vi "LV SCISDK Read List Data.vi"(0 "Path":string, 1 "Buffer Size":u32=1, 2 "handle":u64, 3 "error in (no error)":errorcluster) -> (7 "error out":errorcluster, 8 "buffer out":T1, 9 "handle out":u64, 10 "function return":i32)   [LabVIEW 2021, in "SciSDK_Labview.lvlib"]
doc: "SCISDKLABVIEW_DLL_API int LV_SCISDK_ReadSpectrum(char* Path, TD_SPECTRUM* buffer, void* handle);"
uses:
  SciSDK_Labview.lvlib
panel:
  in  "buffer":T1={"magic"=0, "buffer_size"=0, "samples"=0, "valid_samples"=0, "channels"=0, "data"=[10, 100]}
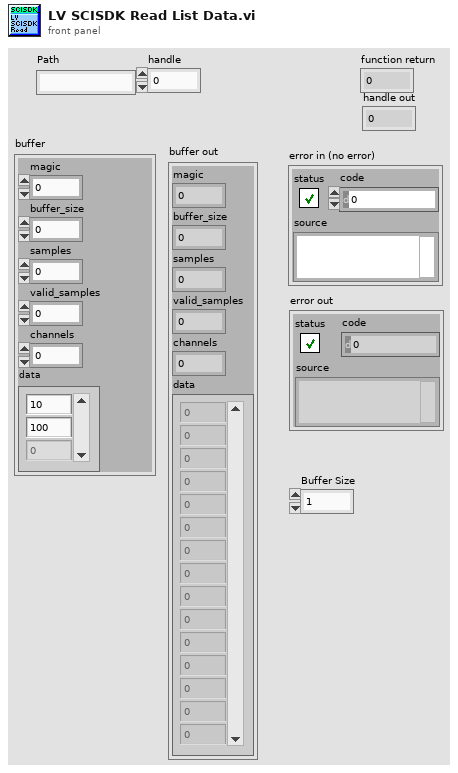
[diagram p1: front panel]
types:
  T1 = cluster{"magic":u32, "buffer_size":u32, "samples":u32, "valid_samples":u32, "channels":u32, "data":i8[]}
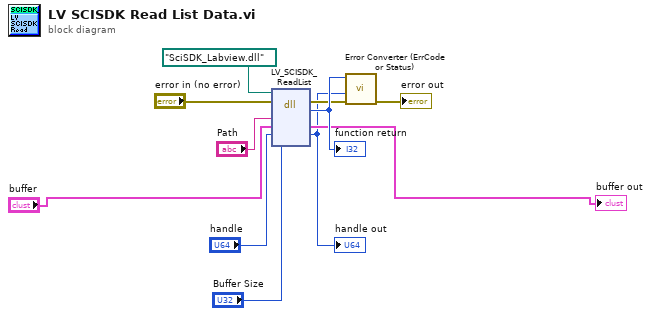
[diagram p0: block diagram]
diagram:
  n1 = dll-call lib="C:/git/scisdk/SciSDK_VC++/x64/Debug/SciSDK_Labview.dll" fn="LV_SCISDK_ReadList"(path in=path "SciSDK_Labview.dll", error in="error in (no error)", "Path"="Path", "buffer"="buffer", "handle"="handle", "buffer_size"="Buffer Size") -> (error out=w7:errorcluster, "return type"=w11:i32, "buffer"=→"buffer out":T1, "handle"=w1:u64)  [unwired: 3 in, 1 out]
  "function return" <- w11
  "handle out" <- w1
  n2 = call "Error Converter (ErrCode or Status).vi"("error in (no error)"=w7, "handle"=w1, "error code"=w11) -> ("error out"=→"error out":errorcluster)  [unwired: 8 in]
